vi "Auto - Turn an Angle.vi"(9 "Auton Cluster In":T2, 11 "Auton State In":i32) -> (1 "Auton Cluster Out":T2, 3 "Auton State Out":i32, 6 "rotation":dbl)   [LabVIEW 2020]
uses:
  TypeDefs/Auton Cluster Typedef.ctl
  Team Code/Robot Global Data.vi
  <vilib>/addons/control/pid/pid.llb/PID (DBL).vi
  <vilib>/addons/control/pid/NI_PID_pid.lvlib
panel:
  in  "PID gains":T1={"proportional gain (Kc)"=0.005, "integral time (Ti, min)"=0.0, "derivative time (Td, min)"=0.0} {"derivative time (Td, min)" format="%.3f"; "integral time (Ti, min)" format="%.3f"; "proportional gain (Kc)" format="%.3f"}
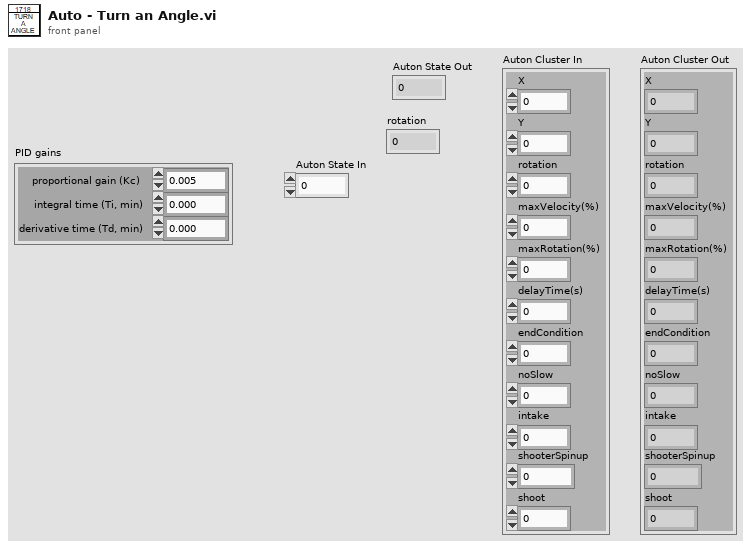
[diagram p1: front panel]
types:
  T1 = cluster{"proportional gain (Kc)":dbl, "integral time (Ti, min)":dbl, "derivative time (Td, min)":dbl}
  T2 = typedef "Auton Cluster Typedef.ctl" = cluster{"rotation":dbl, "maxVelocity(%)":dbl, "delayTime(s)":dbl, "endCondition":dbl, "noSlow":dbl, "intake":dbl, "shooterSpinup":dbl, "shoot":dbl, "X":dbl, "Y":dbl, "maxRotation(%)":dbl}
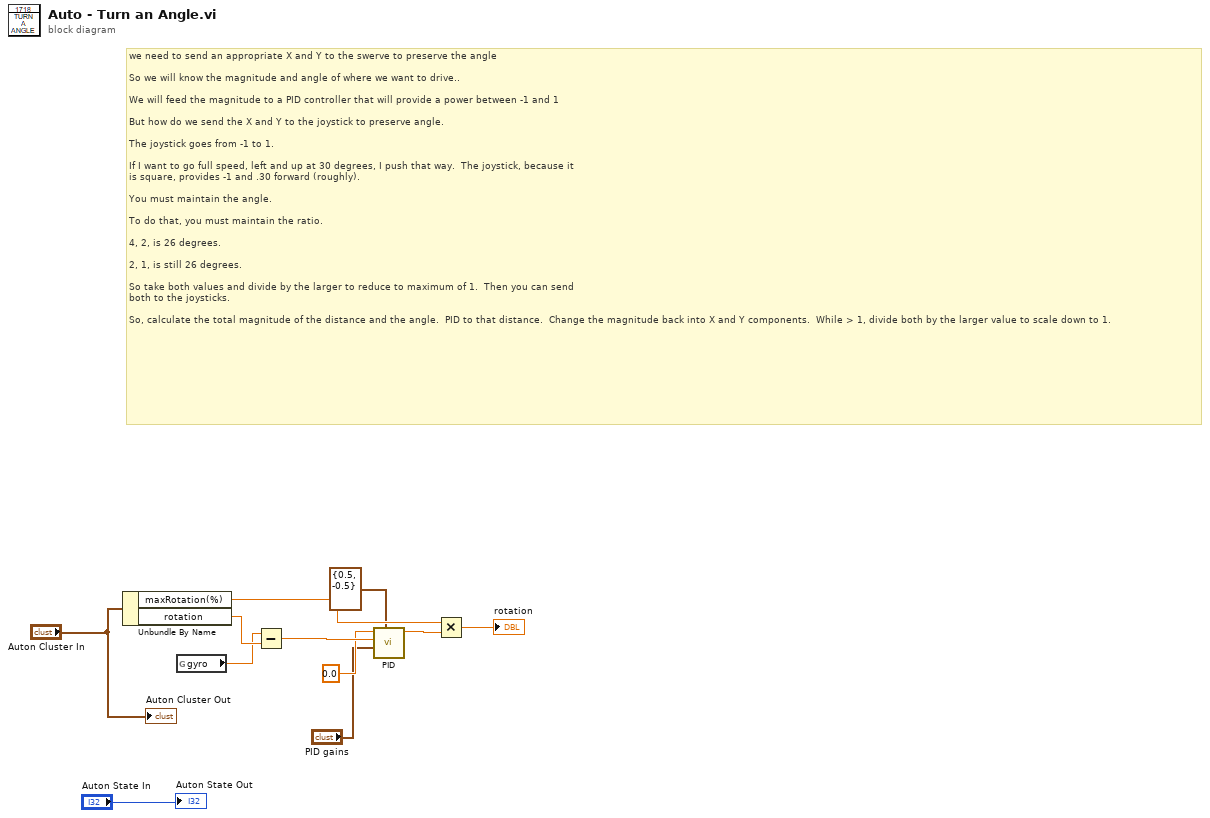
[diagram p0: block diagram]
diagram:
  # "we need to send an appropriate X and Y to the swerve to preserve the angle \n\nSo we will know the magnitude and angle of where we want to drive..\n\nWe will feed the magnitude to a PID controller that will provide a power between -1 and 1\n\nBut how do we send the X and Y to the joystick to preserve angle.\n\nThe joystick goes from -1 to 1.\n\nIf I want to go full speed, left and up at 30 degrees, I push that way.  The joystick, because it\nis square, provides -1 and .30 forward (roughly).\n\nYou must maintain the angle.\n\nTo do that, you must maintain the ratio.\n\n4, 2, is 26 degrees.\n\n2, 1, is still 26 degrees.\n\nSo take both values and divide by the larger to reduce to maximum of 1.  Then you can send\nboth to the joysticks.\n\nSo, calculate the total magnitude of the distance and the angle.  PID to that distance.  Change the magnitude back into X and Y components.  While > 1, divide both by the larger value to scale down to 1."
  n1 = Unbundle By Name("Auton Cluster In") -> ("maxRotation(%)"=w9:dbl, "rotation"=w7:dbl)
  n2 = global read "Robot Global Data.vi" "gyro"() -> (w6:dbl)
  n3 = Subtract(x=w6, y=w7) -> (x-y=w5:dbl)
  n4 = call-poly <vilib>:"PID.vi"("output range"=cluster{"output high":dbl, "output low":dbl} {"output high"=0.5, "output low"=-0.5}, "PID gains"="PID gains", "process variable"=w5, "setpoint"=0.0) -> ("output"=w3:dbl)  [unwired: 6 in, 1 out]
  n5 = Multiply(x=w9, y=w3) -> (x*y=→"rotation":dbl)
  "Auton Cluster Out" <- "Auton Cluster In"
  "Auton State Out" <- "Auton State In"
